vi "LargeMotor.vi"   [LabVIEW 2016, in "Moving Motor.lvrbt"]
uses:
  Moving Motor.lvrbt
  <vilib>/NXT/Block Support/NXT_OutputPort.ctl
  <vilib>/NXT/NXTIO Xnodes/NXTIONodeSubVIs/NXTMoveMotors.vi
  <vilib>/NXT/Subs/LVHSConnector.ctl
  <vilib>/NXT/NXTIO Xnodes/AddressXNode/NXTIOAddress.xnode
  <vilib>/NXT/NXTIO Xnodes/NXTIOXNode/NXTIO.xnode
  <vilib>/NXT/LegoClasses/BrickReference/BrickReference.lvclass
types:
  T1 = typedef "NXT_OutputPort.ctl" = u8
  T2 = typedef "LVHSConnector.ctl" = refnum<class "BrickReference.lvclass">
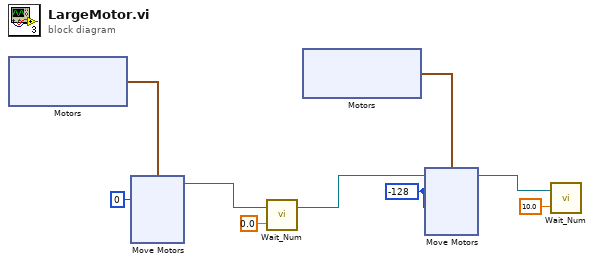
[diagram p0: block diagram]
diagram:
  w3 = i8 -128 ("Power/Speed 1")
  n1 = xnode "Motors"() -> ("Motor"=w9:cluster{"Port":T1, "Port":T1})
  n2 = xnode "Move Motors"("Power/Speed 1"=i8 0, "Motors"=w9) -> ("NXT/EV3"=w7:T2)  [unwired: 2 in]
  n3 = call <vilib>:"Wait_Num.vi"("Time (1 sec)"=sgl 0.0, "NXT/EV3"=w7) -> ("NXT/EV3"=w4:T2)  [unwired: 2 in]
  n4 = xnode "Motors"() -> ("Motor"=w5:cluster{"Port":T1, "Port":T1})
  n5 = xnode "Move Motors"("Power/Speed 2"=w3, "Power/Speed 1"=w3, "Motors"=w5, "NXT/EV3"=w4) -> ("NXT/EV3"=w2:T2)
  n6 = call <vilib>:"Wait_Num.vi"("Time (1 sec)"=sgl 10.0, "NXT/EV3"=w2) -> ()  [unwired: 2 in, 1 out]
